vi "Read XML_Parse Channels.vi"(8 "error in (no error)":errorcluster, 11 "channel429":refnum<k24>[](array[refnum])) -> (0 "error out":errorcluster, 3 "Array":T1[](array[typedef]) {"speed" items=["Auto", "Low", "High"]; "Labels"."scheduleBuildUnit" items=["Millisecond", "Microsecond"]})   [LabVIEW 2016]
uses:
  Controls/Ballard_Channel.ctl
  Controls/Ballard_Label.ctl
  Controls/Ballard_Word.ctl
  Controls/ARINCParam.ctl
  Shared/Controls and Global/TransferType.ctl
  Controls/Channel_direction.ctl
  Controls/Channel Speed.ctl
  C:/Users/Vincent/Desktop/Ballard-Arinc-429-Custom-Device/Source/System Explorer/SubVIs/Parse XML Ballard/Ballard_BTI_XML_Deserializer.dll
  Ballard_BTI_XML_Deserializer.dll
  Ballard Arinc-429 System Explorer.lvlib
  Shared/Ballard Arinc-429 Shared.lvlib
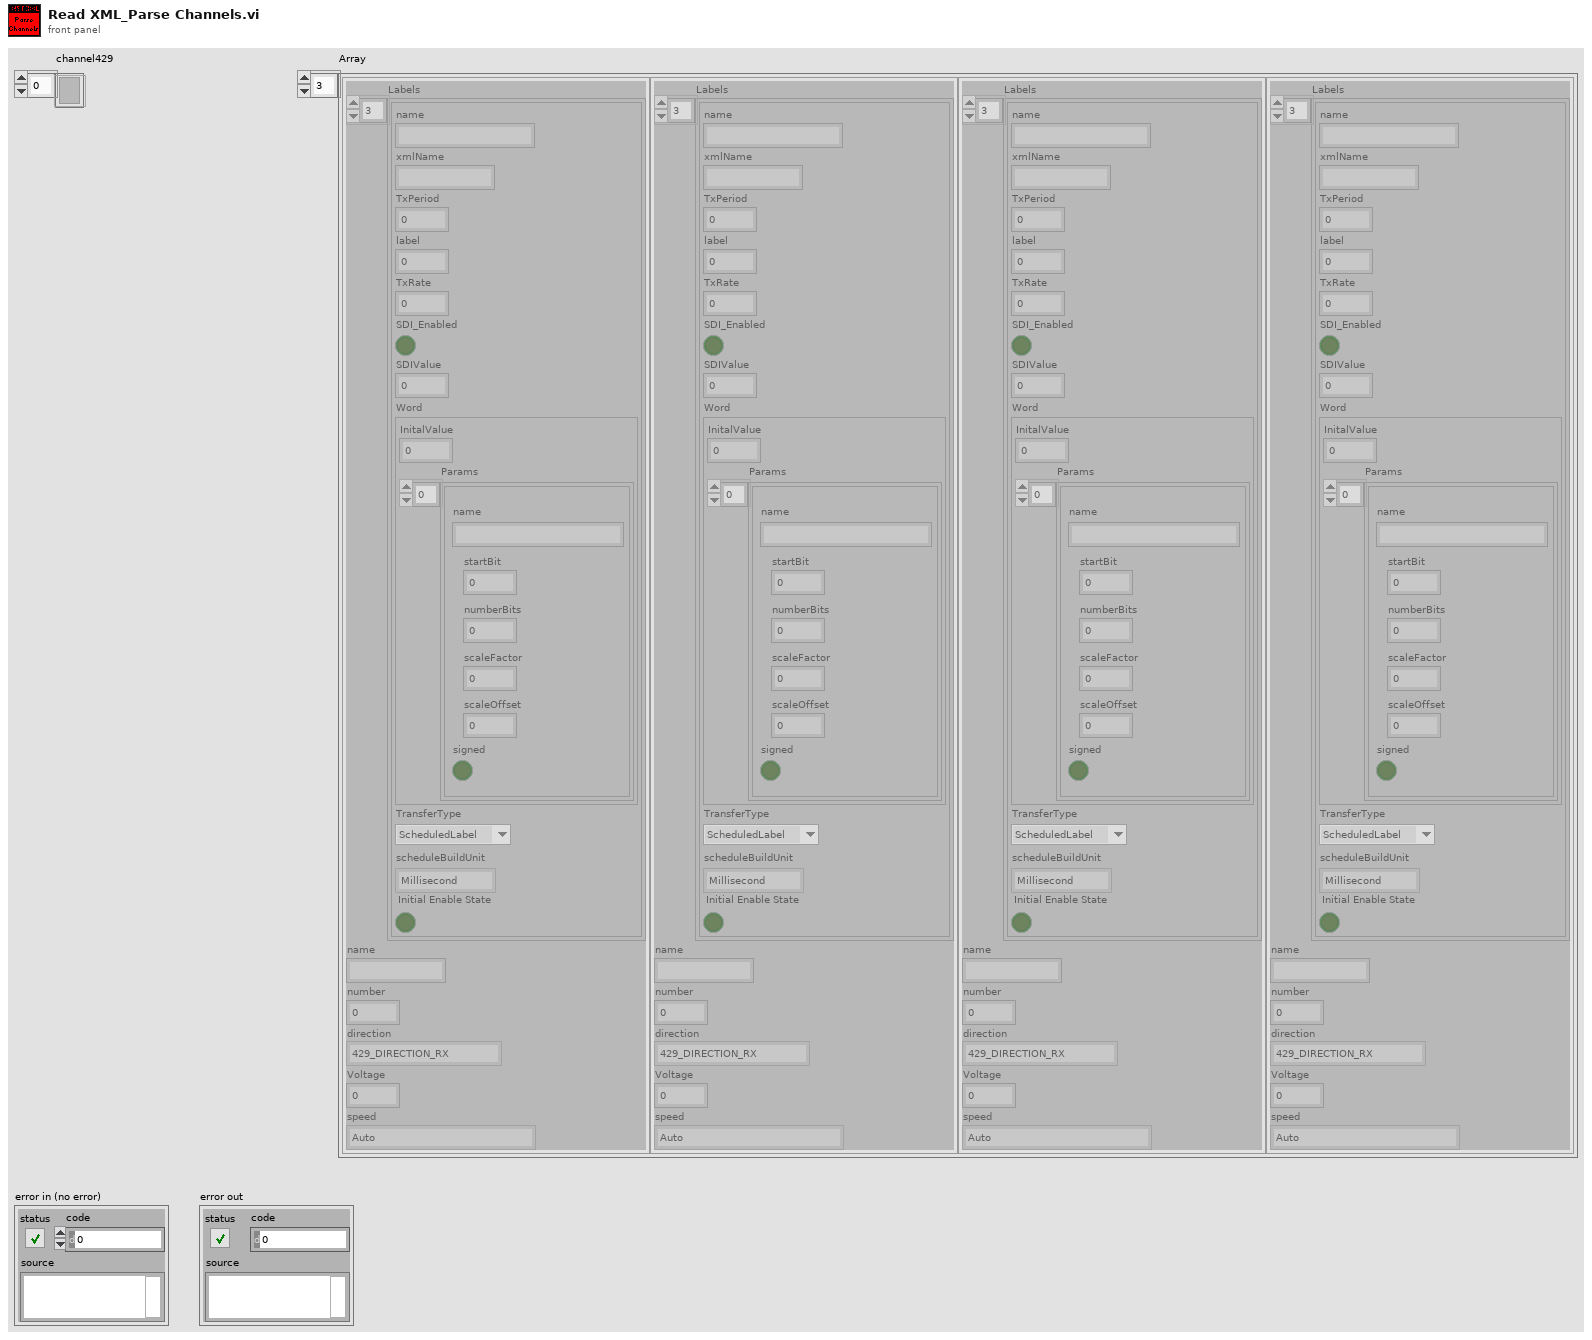
[diagram p1: front panel]
types:
  T1 = typedef "Ballard Arinc-429 System Explorer.lvlib/Ballard_Channel.ctl" = cluster{"Labels":T2[], "name":string, "number":u8, "direction":T6, "Voltage":dbl, "speed":T7}
  T2 = typedef "Ballard Arinc-429 System Explorer.lvlib/Ballard_Label.ctl" = cluster{"name":string, "xmlName":string, "TxPeriod":u32, "label":u32, "TxRate":dbl, "SDI_Enabled":bool, "SDIValue":u8, "Word":T3, "TransferType":T5, "scheduleBuildUnit":i32, "Initial Enable State":bool}
  T3 = typedef "Ballard Arinc-429 System Explorer.lvlib/Ballard_Word.ctl" = cluster{"InitalValue":u32, "Params":T4[]}
  T4 = typedef "Ballard Arinc-429 System Explorer.lvlib/ARINCParam.ctl" = cluster{"name":string, "startBit":i32, "numberBits":i32, "scaleFactor":dbl, "scaleOffset":dbl, "signed":bool}
  T5 = typedef "Ballard Arinc-429 Shared.lvlib/TransferType.ctl" = enum16{"ScheduledLabel", "Acyclic", "Block", "Strobe"}
  T6 = typedef "Ballard Arinc-429 System Explorer.lvlib/Channel_direction.ctl" = enum16{"429_DIRECTION_RX", "429_DIRECTION_TX"}
  T7 = typedef "Ballard Arinc-429 System Explorer.lvlib/Channel Speed.ctl" = i32
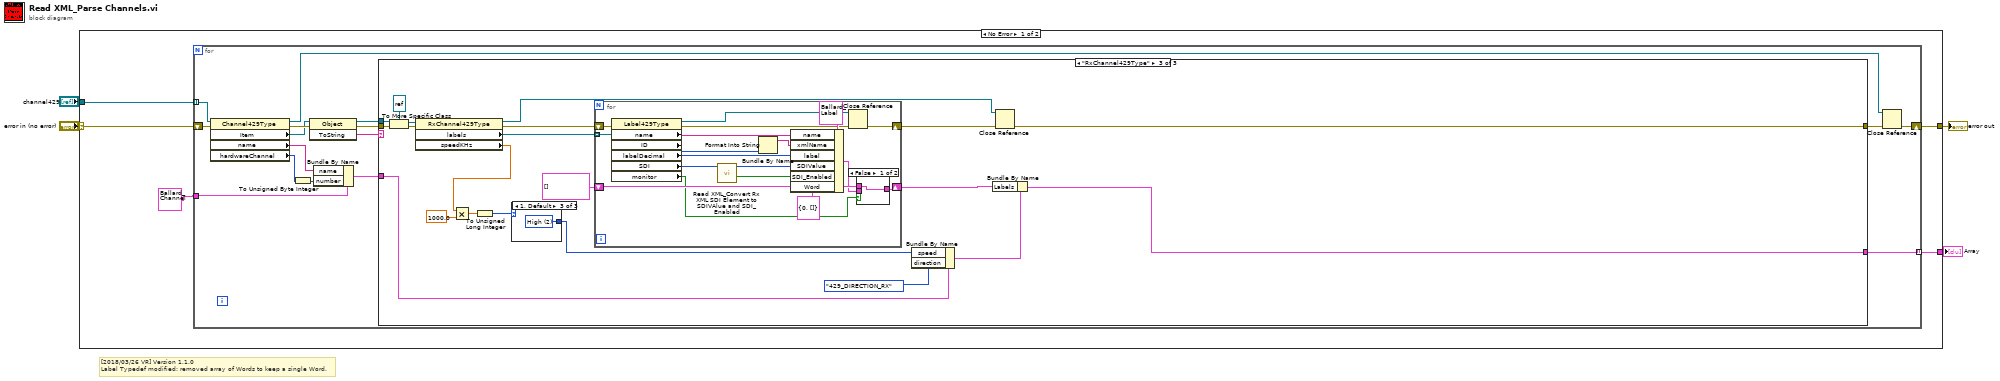
[diagram p0: block diagram]
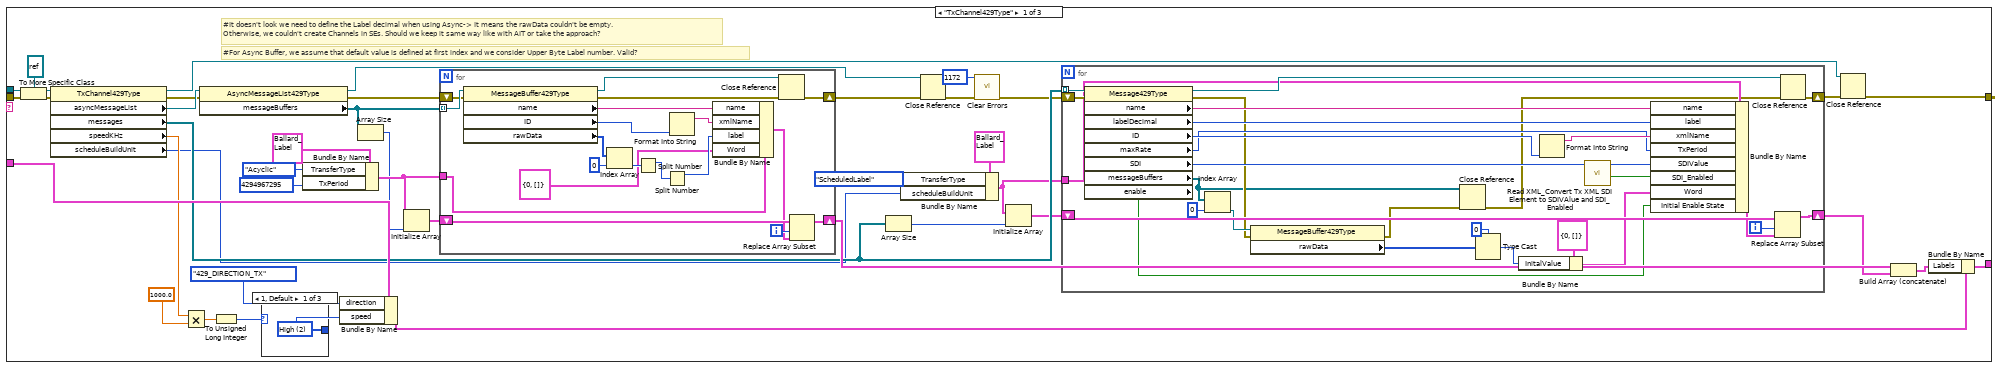
[diagram p2: hidden frame]
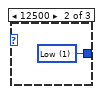
[diagram p3: hidden frame]
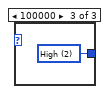
[diagram p4: hidden frame]
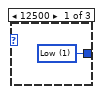
[diagram p6: hidden frame]
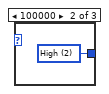
[diagram p7: hidden frame]
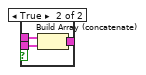
[diagram p8: hidden frame]
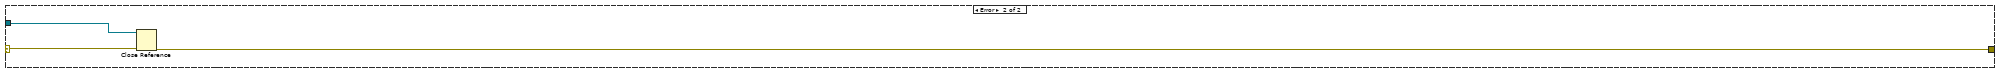
[diagram p9: hidden frame]
diagram:
  # "[2018/03/26 VR] Version 1.1.0\nLabel Typedef modified: removed array of Words to keep a single Word."
  n1 = case shown="No Error" "error in (no error)" {
    selector: "error in (no error)" -> [w5 w168]
    tunnel: [w9 _] -> w4
    tunnel: [w7 w167] -> w3
    tunnel: "channel429" -> [w6 w169]
    frame No Error {
      n2 = for {
        tunnel: w6 -> [w25] mode=indexing
        shift-right: [w11] -> w7
        shift-left: w5 -> [w22]
        tunnel: T1 {"Labels"=[], "name"="", "number"=0, "direction"=enum."429_DIRECTION_RX", "Voltage"=0.0, "speed"=0} ("channel") -> [w18]
        tunnel: [w13] -> w9 mode=indexing
        n3 = property class="Channel429Type"(reference=w25, error in=w22) -> (reference out=w10:refnum<k24>, error out=w21:errorcluster, "Item"=w19:refnum<k24>, "name"=w17:string, "hardwareChannel"=w16:i32)
        n4 = To Unsigned Byte Integer(number=w16) -> (unsigned 8bit integer=w15:u8)
        n5 = invoke class="Object" method="ToString"(reference=w19, error in=w21) -> (reference out=w23:refnum<k24>, error out=w20:errorcluster, "ToString"=w24:string)  [unwired: 1 in]
        n6 = Bundle By Name(cluster=w18, "name"=w17, "number"=w15) -> (w14:T1)
        n7 = case shown="\"RxChannel429Type\"" w24 {
          tunnel: w23 -> [w67 _ w141]
          tunnel: w20 -> [w66 w120 w140]
          tunnel: [w54 w120 w127] -> w12
          tunnel: w14 -> [w52 w119 w130]
          tunnel: [w40 w119 w132] -> w13
          frame "TxChannel429Type" {
            # "#For Async Buffer, we assume that default value is defined at first index and we consider Upper Byte Label number. Valid?"
            # "#It doesn't look we need to define the Label decimal when using Async-> It means the rawData couldn't be empty.\nOtherwise, we couldn't create Channels in SEs. Should we keep it same way like with AIT or take the approach?"
            n8 = To More Specific Class(target class=refnum<k24> refnum, reference=w67, error in=w66) -> (specific class reference=w63:refnum<k24>, error out=w64:errorcluster)
            n9 = property class="TxChannel429Type"(reference=w63, error in=w64) -> (reference out=w55:refnum<k24>, error out=w61:errorcluster, "asyncMessageList"=w62:refnum<k24>, "messages"=w38:refnum<k24>[], "speedKHz"=w33:dbl, "scheduleBuildUnit"=w29:i32)
            n10 = Multiply(x=w33, y=1000.0) -> (x*y=w34:dbl)
            n11 = property class="AsyncMessageList429Type"(reference=w62, error in=w61) -> (reference out=w57:refnum<k24>, error out=w60:errorcluster, "messageBuffers"=w48:refnum<k24>[])
            n12 = To Unsigned Long Integer(number=w34) -> (unsigned 32bit integer=w31:u32)
            n13 = case shown="1, Default" w31 {
              tunnel: [w68 w69 w70] -> w30
              frame 1, Default {
                w68 = T7 2 items=["Auto", "Low", "High"] ("speed")
              }
              frame 12500 {
                w69 = T7 1 items=["Auto", "Low", "High"] ("speed")
              }
              frame 100000 {
                w70 = T7 2 items=["Auto", "Low", "High"] ("speed")
              }
            }
            n14 = Bundle By Name(cluster=T2 {"name"="", "xmlName"="", "TxPeriod"=0, "label"=0, "TxRate"=0.0, "SDI_Enabled"=FALSE, "SDIValue"=0, "Word"={"InitalValue"=0, "Params"=[]}, "TransferType"=enum."ScheduledLabel", "scheduleBuildUnit"=0, "Initial Enable State"=FALSE} ("Label"), "TransferType"=TransferType."Acyclic", "TxPeriod"=u32 4294967295) -> (w49:T2)
            n15 = Bundle By Name(cluster=w52, "direction"=Channel_direction."429_DIRECTION_TX", "speed"=w30) -> (w44:T1)
            n16 = Array Size(array=w48) -> (size(s)=w47:i32)
            n17 = Initialize Array(w49, w47) -> (w46:T2[])
            n18 = for {
              tunnel: w48 -> [w118] mode=indexing
              shift-right: [w114] -> w59
              shift-left: w60 -> [w117]
              tunnel: w49 -> [w109]
              shift-right: [w112] -> w43
              shift-left: w46 -> [w113]
              i -> [w111]
              n19 = property class="MessageBuffer429Type"(reference=w118, error in=w117) -> (reference out=w115:refnum<k24>, error out=w116:errorcluster, "name"=w108:string, "ID"=w107:i32, "rawData"=w105:u8[])
              n20 = Index Array(array=w105, index=0) -> (element=w103:u8)
              n21 = Split Number(x=w103) -> (hi(x)=w102:u8)  [unwired: 1 out]
              n22 = Split Number(x=w102) -> (hi(x)=w101:u8)  [unwired: 1 out]
              n23 = Format Into String(w107) -> (resulting string=w106:string)  [unwired: 3 in, 1 out]
              n24 = Bundle By Name(cluster=w109, "name"=w108, "xmlName"=w106, "label"=w101, "Word"=T3 {"InitalValue"=0, "Params"=[]}) -> (w110:T2)
              n25 = Close Reference(reference=w115, error in (no error)=w116) -> (error out=w114:errorcluster)
              n26 = Replace Array Subset(array=w113, new element=w110, index=w111) -> (w112:T2[])
            }
            n27 = Array Size(array=w38) -> (size(s)=w36:i32)
            n28 = Bundle By Name(cluster=T2 {"name"="", "xmlName"="", "TxPeriod"=0, "label"=0, "TxRate"=0.0, "SDI_Enabled"=FALSE, "SDIValue"=0, "Word"={"InitalValue"=0, "Params"=[]}, "TransferType"=enum."ScheduledLabel", "scheduleBuildUnit"=0, "Initial Enable State"=FALSE} ("Label"), "TransferType"=TransferType."ScheduledLabel", "scheduleBuildUnit"=w29) -> (w37:T2)
            n29 = Close Reference(reference=w57, error in (no error)=w59) -> (error out=w58:errorcluster)
            n30 = call <vilib>:"Clear Errors.vi"("error in (no error)"=w58, "specific error code to clear (0: all)"=1172) -> ("error out"=w27:errorcluster)  [unwired: 4 in, 1 out]
            n31 = Initialize Array(w37, w36) -> (w35:T2[])
            n32 = for {
              tunnel: w38 -> [w99] mode=indexing
              shift-right: [w97] -> w56
              shift-left: w27 -> [w98]
              tunnel: w37 -> [w92]
              shift-right: [w95] -> w28
              shift-left: w35 -> [w93]
              i -> [w94]
              n33 = property class="Message429Type"(reference=w99, error in=w98) -> (reference out=w96:refnum<k24>, error out=w80:errorcluster, "name"=w91:string, "labelDecimal"=w89:i32, "ID"=w88:i32, "maxRate"=w86:i32, "SDI"=w85:i32, "messageBuffers"=w79:refnum<k24>[], "enable"=w71:bool)
              n34 = Index Array(array=w79, index=0) -> (element=w81:refnum<k24>)
              n35 = property class="MessageBuffer429Type"(reference=w81, error in=w80) -> (error out=w78:errorcluster, "rawData"=w73:u8[])  [unwired: 1 out]
              n36 = Close Reference(reference=w79, error in (no error)=w78) -> (error out=w77:errorcluster)
              n37 = Type Cast(type=u32 0, x=w73) -> (*(type *) &x=w74:u32)
              n38 = Bundle By Name(cluster=T3 {"InitalValue"=0, "Params"=[]} ("Word"), "InitalValue"=w74) -> (w72:T3)
              n39 = Format Into String(w88) -> (resulting string=w87:string)  [unwired: 3 in, 1 out]
              n40 = call "Read XML_Convert Tx XML SDI Element to SDIVAlue and SDI_Enabled.vi"("SDI"=w85) -> ("SDI_Enabled"=w83:bool, "SDIValue"=w84:u8)  [unwired: 9 in]
              n41 = Bundle By Name(cluster=w92, "name"=w91, "label"=w89, "xmlName"=w87, "TxPeriod"=w86, "SDIValue"=w84, "SDI_Enabled"=w83, "Word"=w72, "Initial Enable State"=w71) -> (w90:T2)
              n42 = Replace Array Subset(array=w93, new element=w90, index=w94) -> (w95:T2[])
              n43 = Close Reference(reference=w96, error in (no error)=w77) -> (error out=w97:errorcluster)
            }
            n44 = Close Reference(reference=w55, error in (no error)=w56) -> (error out=w54:errorcluster)
            n45 = Build Array (concatenate)(w43, w28) -> (w39:T2[])
            n46 = Bundle By Name(cluster=w44, "Labels"=w39) -> (w40:T1)
          }
          frame "False", Default {
          }
          frame "RxChannel429Type" {
            n47 = To More Specific Class(target class=refnum<k24> refnum, reference=w141, error in=w140) -> (specific class reference=w137:refnum<k24>, error out=w138:errorcluster)
            n48 = property class="RxChannel429Type"(reference=w137, error in=w138) -> (reference out=w126:refnum<k24>, error out=w135:errorcluster, "labels"=w136:refnum<k24>[], "speedKHz"=w123:dbl)
            n49 = Multiply(x=w123, y=1000.0) -> (x*y=w125:dbl)
            n50 = To Unsigned Long Integer(number=w125) -> (unsigned 32bit integer=w122:u32)
            n51 = case shown="1, Default" w122 {
              tunnel: [w142 w143 w144] -> w121
              frame 12500 {
                w142 = T7 1 items=["Auto", "Low", "High"] ("speed")
              }
              frame 100000 {
                w143 = T7 2 items=["Auto", "Low", "High"] ("speed")
              }
              frame 1, Default {
                w144 = T7 2 items=["Auto", "Low", "High"] ("speed")
              }
            }
            n52 = for {
              tunnel: w136 -> [w162] mode=indexing
              shift-right: [w151] -> w128
              shift-left: w135 -> [w161]
              shift-right: [w159] -> w131
              shift-left: T2[] [] ("Labels") -> [w160]
              n53 = property class="Label429Type"(reference=w162, error in=w161) -> (reference out=w150:refnum<k24>, error out=w152:errorcluster, "name"=w154:string, "ID"=w155:i32, "labelDecimal"=w157:i32, "SDI"=w149:i32, "monitor"=w146:bool)
              n54 = call "Read XML_Convert Rx XML SDI Element to SDIVAlue and SDI_Enabled.vi"("SDI"=w149) -> ("SDI_Enabled"=w147:bool, "SDIValue"=w148:u8)  [unwired: 9 in]
              n55 = Format Into String(w155) -> (resulting string=w156:string)  [unwired: 3 in, 1 out]
              n56 = Bundle By Name(cluster=T2 {"name"="", "xmlName"="", "TxPeriod"=0, "label"=0, "TxRate"=0.0, "SDI_Enabled"=FALSE, "SDIValue"=0, "Word"={"InitalValue"=0, "Params"=[]}, "TransferType"=enum."ScheduledLabel", "scheduleBuildUnit"=0, "Initial Enable State"=FALSE} ("TxScheduledLabel"), "name"=w154, "xmlName"=w156, "label"=w157, "SDIValue"=w148, "SDI_Enabled"=w147, "Word"=T3 {"InitalValue"=0, "Params"=[]}) -> (w153:T2)
              n57 = Close Reference(reference=w150, error in (no error)=w152) -> (error out=w151:errorcluster)
              n58 = case shown="False" w146 {
                tunnel: w160 -> [w163 w166]
                tunnel: [w163 w165] -> w159
                tunnel: w153 -> [_ w164]
                frame False {
                }
                frame True {
                  n59 = Build Array (concatenate)(w166, w164) -> (w165:T2[])
                }
              }
            }
            n60 = Bundle By Name(cluster=w130, "speed"=w121, "direction"=Channel_direction."429_DIRECTION_RX") -> (w133:T1)
            n61 = Bundle By Name(cluster=w133, "Labels"=w131) -> (w132:T1)
            n62 = Close Reference(reference=w126, error in (no error)=w128) -> (error out=w127:errorcluster)
          }
        }
        n63 = Close Reference(reference=w10, error in (no error)=w12) -> (error out=w11:errorcluster)
      }
    }
    frame Error {
      n64 = Close Reference(reference=w169, error in (no error)=w168) -> (error out=w167:errorcluster)
    }
  }
  "Array" <- w4
  "error out" <- w3
